vi "Periodic Tasks.vi"(8 "error in":errorcluster) -> ()   [LabVIEW 2020]
doc: "This VI runs in parallel to other tasks. It can contain as many user-defined periodic loops as you need. These can carry out PID or other sorts of timed response."
uses:
  <vilib>/Rock Robotics/WPI/DriverStation/WPI_DriverStationRobotMode2.ctl
  <vilib>/Rock Robotics/WPI/ThirdParty/Phoenix-LabVIEW/Motor Controller/Controls/CTRE_Phoenix_MotorControl_ControlMode.ctl
  <vilib>/Rock Robotics/WPI/Utilities/WPI_GetSetVariantRefNum.vi
  <vilib>/Rock Robotics/Network Tables/NT Write Numeric Array.vi
  Robot Global Data.vi
  <vilib>/Rock Robotics/Network Tables/NT Write Boolean Array.vi
  <vilib>/Rock Robotics/Network Tables/NT Write Boolean.vi
  <vilib>/Rock Robotics/WPI/RobotDrive/WPI_RobotDriveArcadeDrive_Standard(NoSaturation).vi
panel:
  out "Shooter Motor Outtake":bool
  out "Shooter Motor Intake":bool
  out "Conveyor Motor Outtake":bool
  out "Conveyor Motor Intake":bool
  out "Grabber Motor Intake":bool
  out "Grabber Motor Outtake":bool
  out "Slow Speed On":bool
  out "Backwards On":bool
  # "s"
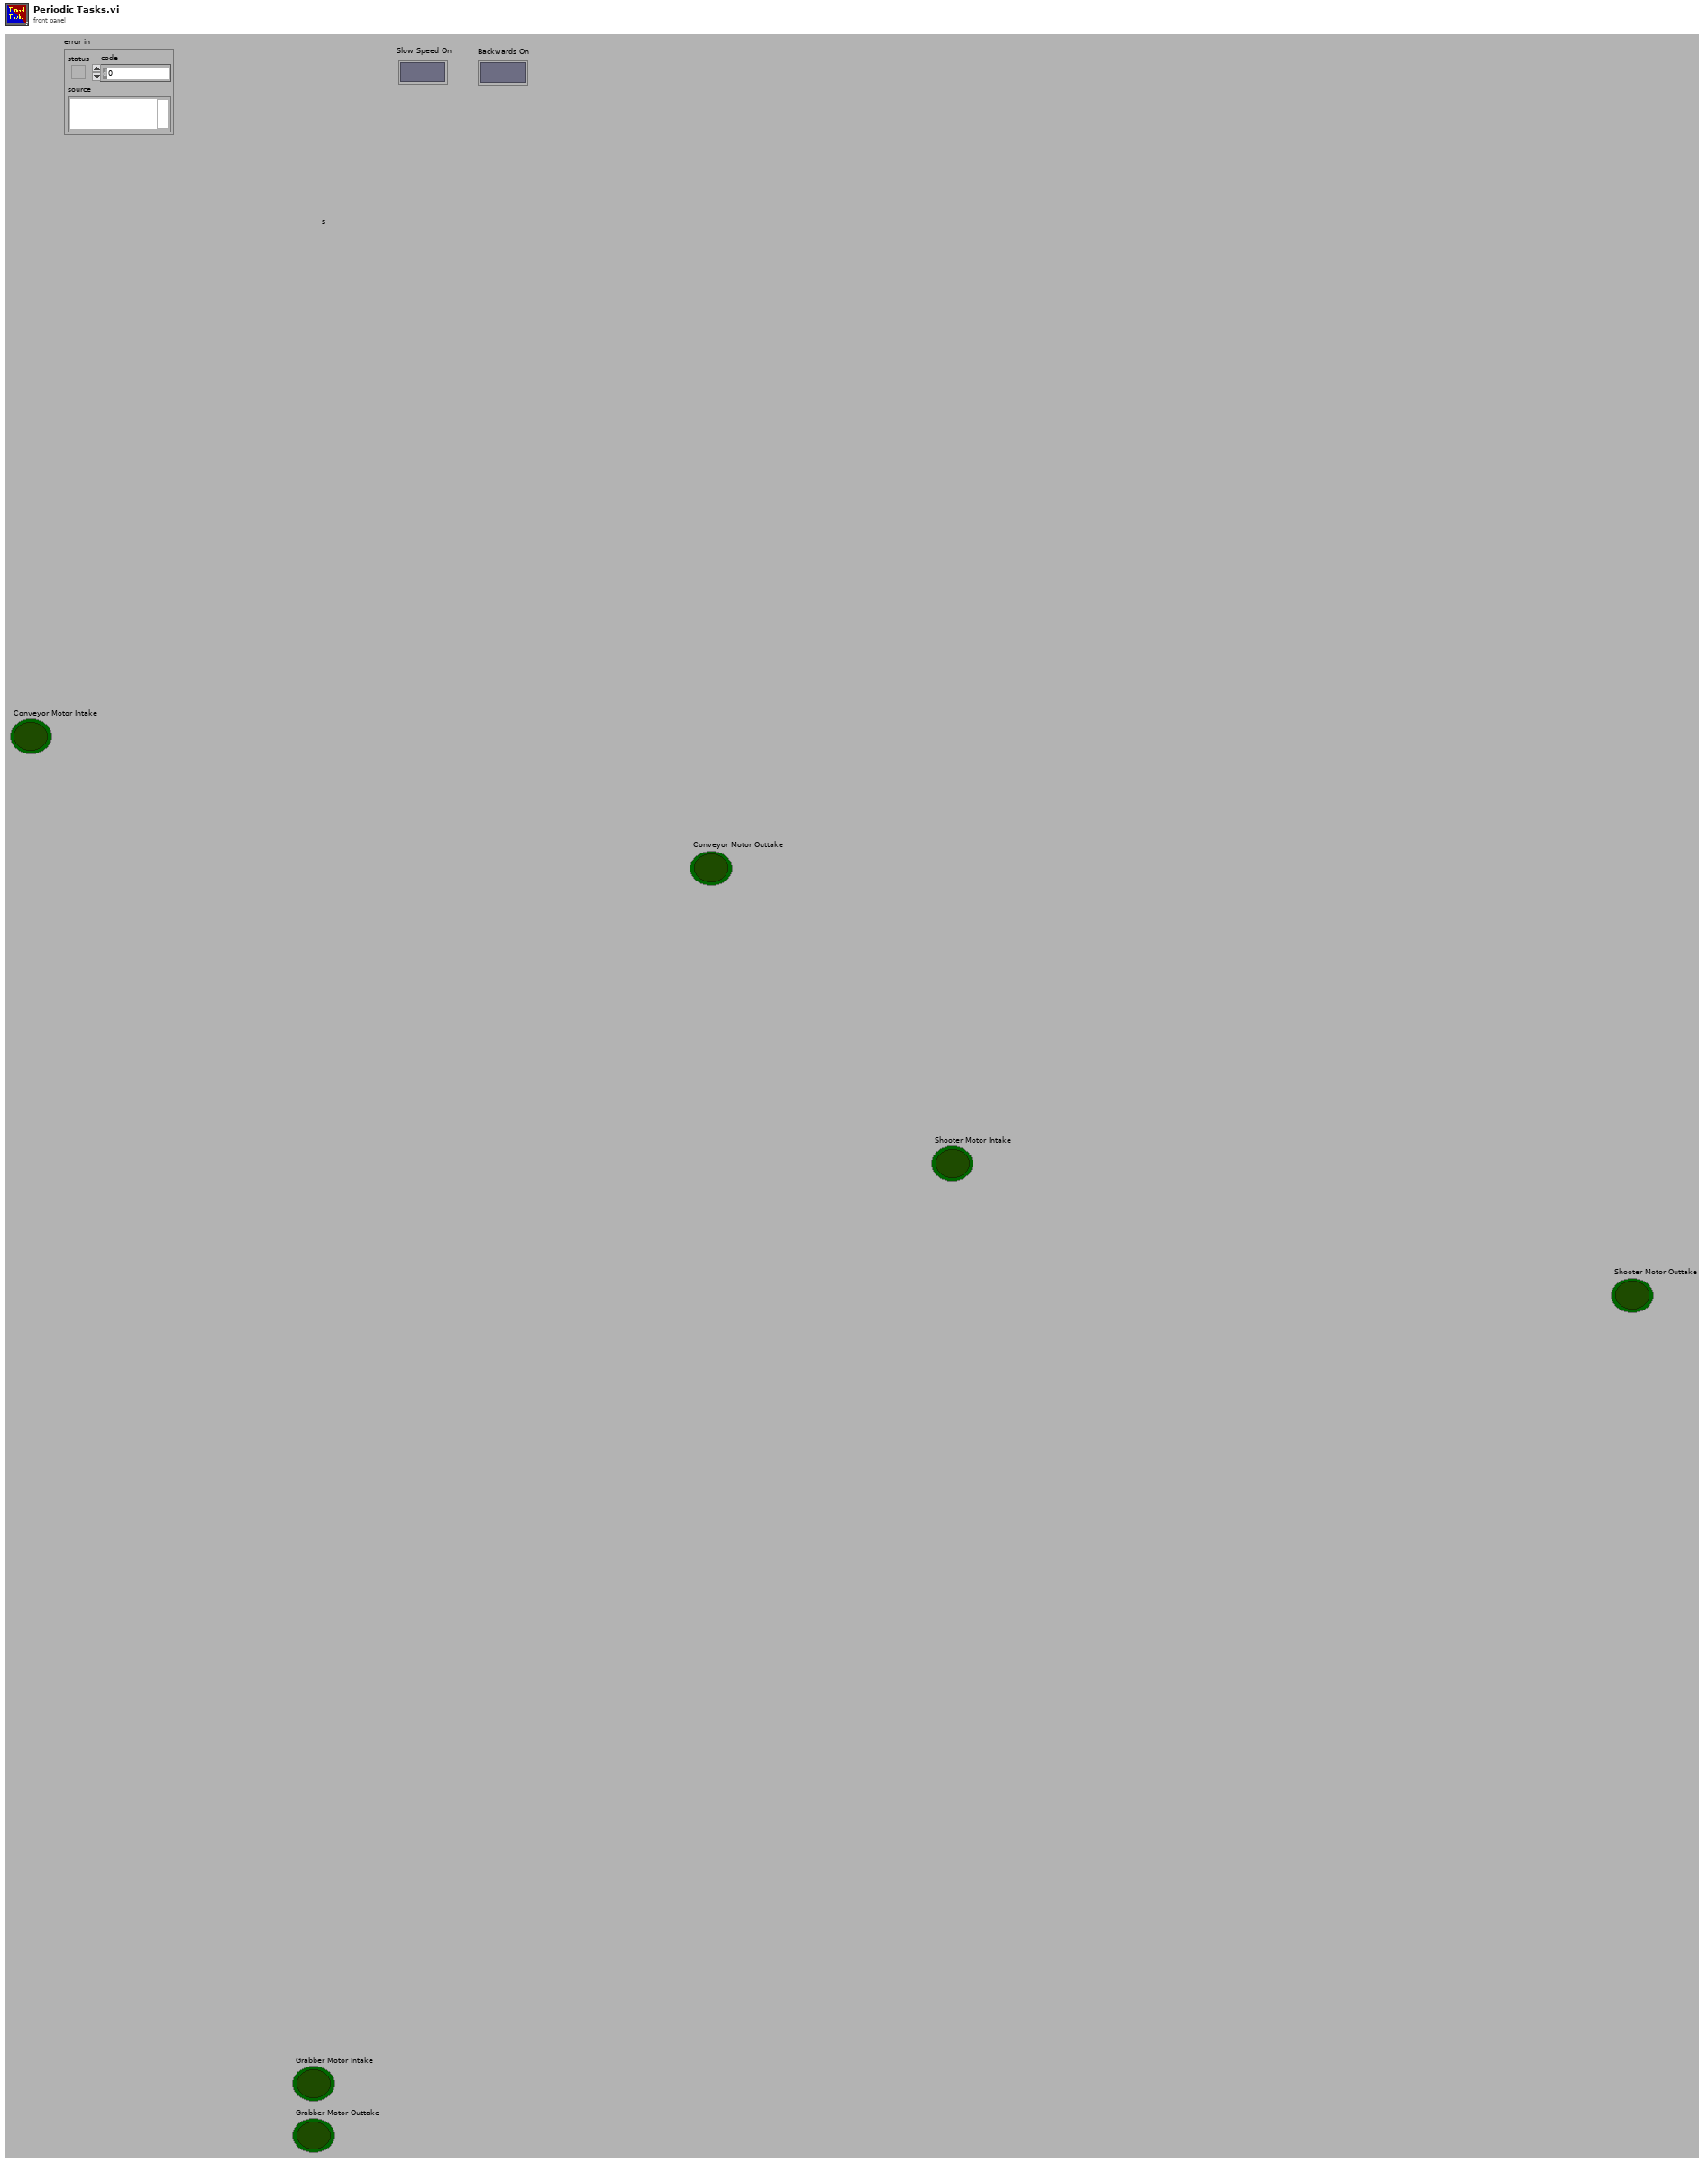
[diagram p1: front panel]
types:
  T1 = typedef "WPI_MotorControlDeviceRef.ctl" = cluster{"DeviceStatus":errorcluster, "Type":T2, "PWM":cluster{"PWM Channel":T3, "DeadBand":T4}, "CAN":cluster{"Device Number":u8, "SetOutput VI Ref":variant, "GetOutput VI Ref":variant, "Enable VI Ref":variant, "Disable VI Ref":variant, "Data":variant}, "Invert":bool, "DIO PWM":cluster{"PWM \"Enable\" Channel":T3, "DIOChannel":T5, "PWM Rate":dbl}}
  T2 = typedef "WPI_MotorControlType.ctl" = enum16{"PWM", "CAN", "DIO PWM"}
  T3 = typedef "FPGA_DIOPWMChannel.ctl" = enum8{"PWM 0", "PWM 1", "PWM 2", "PWM 3", "PWM 4", "PWM 5", "PWM 6", "PWM 7", "PWM 8", "PWM 9", "PWM MXP 0", "PWM MXP 1", "PWM MXP 2", "PWM MXP 3", "PWM MXP 4", "PWM MXP 5", "PWM MXP 6", "PWM MXP 7", "PWM MXP 8", "PWM MXP 9", "Invalid"}
  T4 = typedef "WPI_PWMDeadband.ctl" = cluster{"Name":string, "maxPositivePwm":i32, "minPositivePwm":i32, "centerPwm":i32, "maxNegativePwm":i32, "minNegativePwm":i32, "angularRange":u16}
  T5 = typedef "FPGA_DIOChannel.ctl" = enum8{"DIO 0", "DIO 1", "DIO 2", "DIO 3", "DIO 4", "DIO 5", "DIO 6", "DIO 7", "DIO 8", "DIO 9", "DIO MXP 0", "DIO MXP 1", "DIO MXP 2", "DIO MXP 3", "DIO MXP 4", "DIO MXP 5", "DIO MXP 6", "DIO MXP 7", "DIO MXP 8", "DIO MXP 9", "DIO MXP 10", "DIO MXP 11", "DIO MXP 12", "DIO MXP 13", "DIO MXP 14", "DIO MXP 15", "SPI Port CS1", "SPI Port CS2", "SPI Port CS3", "SPI Port MISO", "SPI Port MOSI", "Invalid"}
  T6 = typedef "WPI_JoystickDevRef.ctl" = cluster{"Device":T7}
  T7 = typedef "WPI_JoystickDeviceEnum.ctl" = enum16{"USB 0", "USB 1", "USB 2", "USB 3", "USB 4", "USB 5"}
  T8 = typedef "WPI_RobotDriveDevRef.ctl" = cluster{"DevStatus":errorcluster, "Motors[]":T1[], "Square Inputs":bool, "Max Output":dbl}
  T9 = typedef "WPI_DriverStationRobotMode2.ctl" = enum16{"Autonomous Disabled", "Autonomous Enabled", "Teleop Disabled", "Teleop Enabled", "Disconnected", "Finish", "Test Disabled", "Test Enabled", "Emergency Stopped"}
  T10 = typedef "CTRE_Phoenix_MotorControl_ControlMode.ctl" = u16
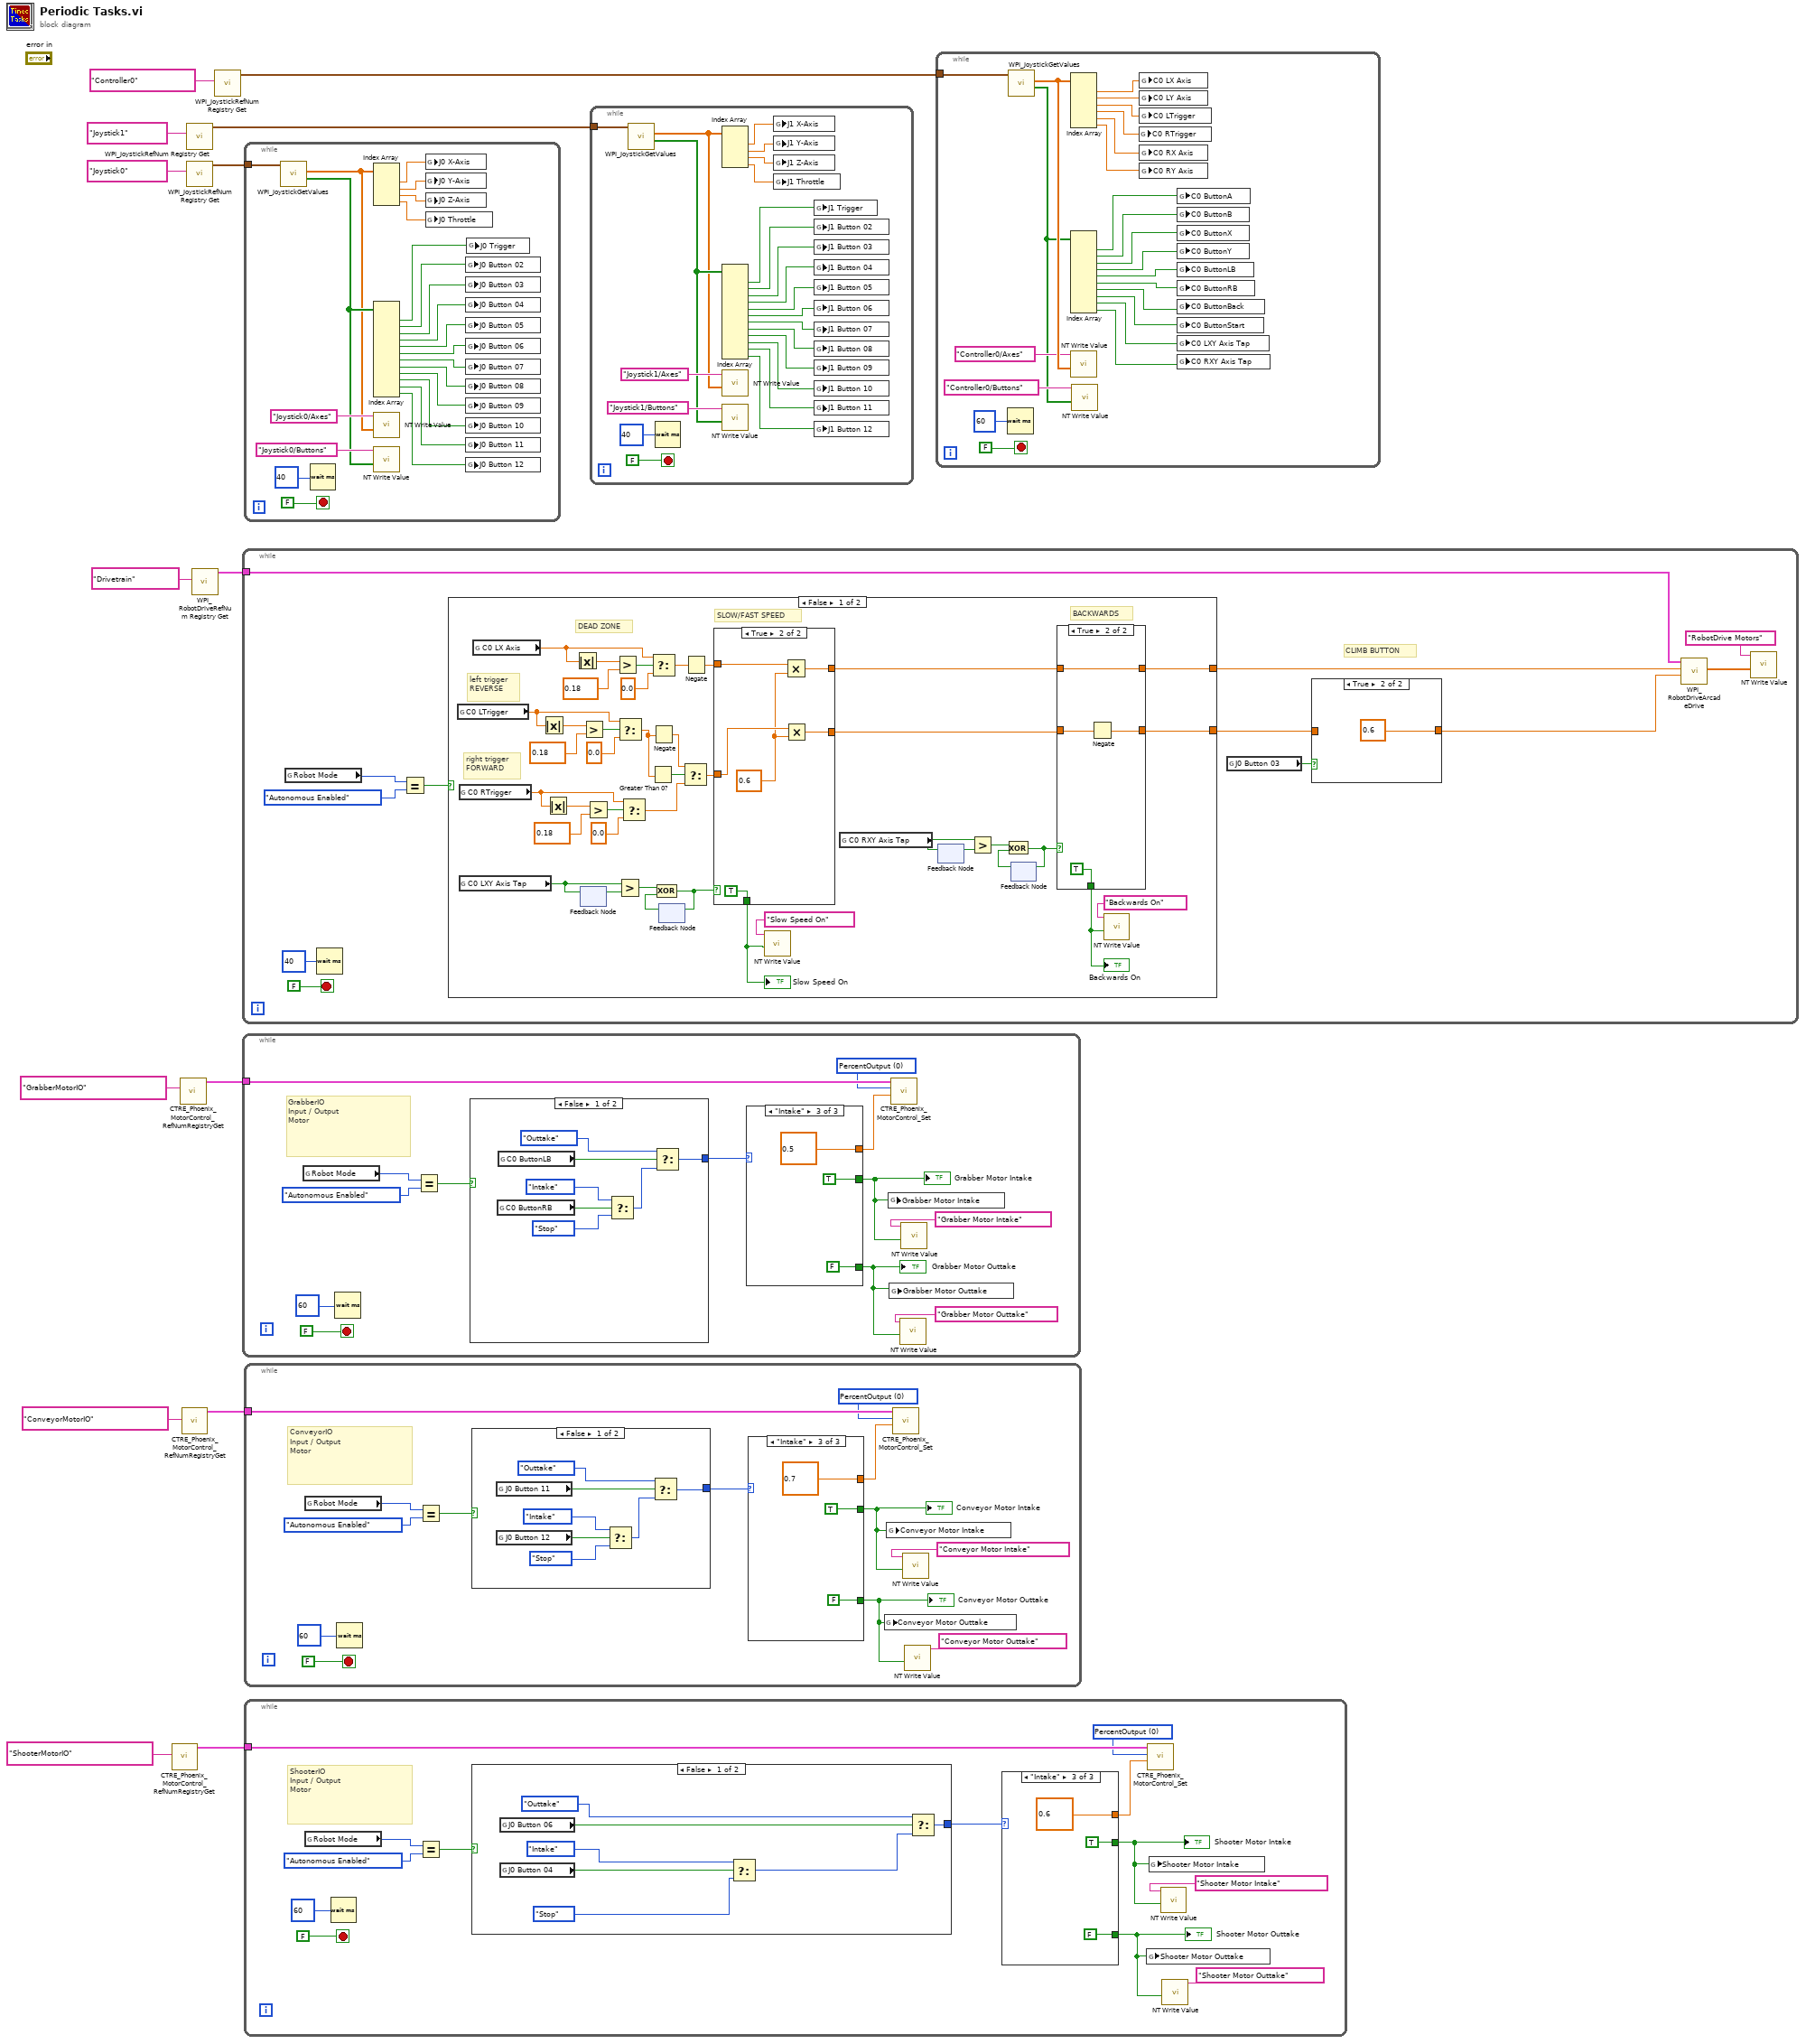
[diagram p0: block diagram]
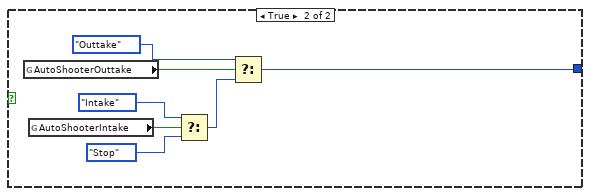
[diagram p2: hidden frame]
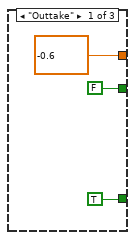
[diagram p3: hidden frame]
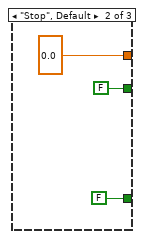
[diagram p4: hidden frame]
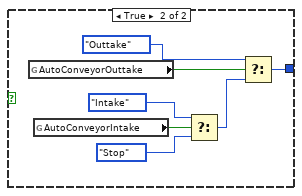
[diagram p5: hidden frame]
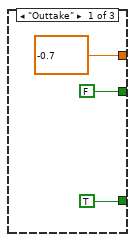
[diagram p6: hidden frame]
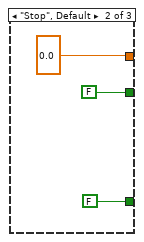
[diagram p7: hidden frame]
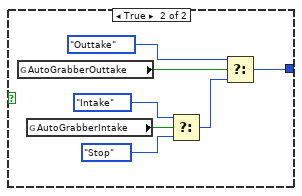
[diagram p8: hidden frame]
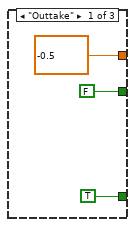
[diagram p9: hidden frame]
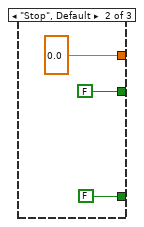
[diagram p10: hidden frame]
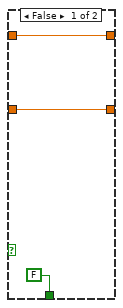
[diagram p12: hidden frame]
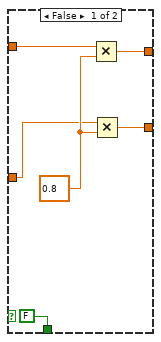
[diagram p13: hidden frame]
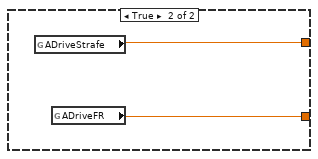
[diagram p14: hidden frame]
diagram:
  n1 = call <vilib>:"CTRE_Phoenix_MotorControl_RefNumRegistryGet.vi"("refnum name"="ShooterMotorIO") -> ("PhoenixMotorControlDevRef"=w2:T1)  [unwired: 9 in, 1 out]
  n2 = call <vilib>:"CTRE_Phoenix_MotorControl_RefNumRegistryGet.vi"("refnum name"="GrabberMotorIO") -> ("PhoenixMotorControlDevRef"=w7:T1)  [unwired: 9 in, 1 out]
  n3 = call <vilib>:"CTRE_Phoenix_MotorControl_RefNumRegistryGet.vi"("refnum name"="ConveyorMotorIO") -> ("PhoenixMotorControlDevRef"=w3:T1)  [unwired: 9 in, 1 out]
  n4 = call <vilib>:"WPI_JoystickRefNum Registry Get.vi"("refnum name"="Joystick1") -> ("JoystickDevRef"=w10:T6)  [unwired: 1 in, 9 out]
  n5 = call <vilib>:"WPI_JoystickRefNum Registry Get.vi"("refnum name"="Joystick0") -> ("JoystickDevRef"=w12:T6)  [unwired: 1 in, 9 out]
  n6 = call <vilib>:"WPI_RobotDriveRefNum Registry Get.vi"("refnum name"="Drivetrain") -> ("RobotDriveDevRef"=w9:T8)  [unwired: 1 in, 9 out]
  n7 = call <vilib>:"WPI_JoystickRefNum Registry Get.vi"("refnum name"="Controller0") -> ("JoystickDevRef"=w5:T6)  [unwired: 1 in, 9 out]
  n8 = while {
    tunnel: w9 -> [w18]
    stop <- FALSE stop-if-true
    # "CLIMB BUTTON"
    n9 = global read "Robot Global Data.vi" "Robot Mode"() -> (w25:T9)
    n10 = Wait (ms)(milliseconds to wait=u32 40) -> ()  [unwired: 1 out]
    n11 = Equal?(x=w25, y=WPI_DriverStationRobotMode2."Autonomous Enabled") -> (x = y?=w23:bool)
    n12 = case shown="False" w23 {
      tunnel: [w43 w88] -> w20
      tunnel: [w42 w89] -> w16
      frame False {
        # "right trigger FORWARD"
        # "left trigger REVERSE"
        # "DEAD ZONE"
        # "BACKWARDS"
        # "SLOW/FAST SPEED"
        n13 = global read "Robot Global Data.vi" "C0 LTrigger"() -> (w53:dbl)
        n14 = global read "Robot Global Data.vi" "C0 RTrigger"() -> (w34:dbl)
        n15 = global read "Robot Global Data.vi" "C0 LXY Axis Tap"() -> (w51:bool)
        n16 = global read "Robot Global Data.vi" "C0 LX Axis"() -> (w54:dbl)
        n17 = Absolute Value(x=w53) -> (abs(x)=w64:dbl)
        n18 = Absolute Value(x=w34) -> (abs(x)=w37:dbl)
        n19 = Absolute Value(x=w54) -> (abs(x)=w62:dbl)
        n20 = feedback #1() -> (w67:bool)  [unwired: 1 in]
        n21 = feedback-in #1(w51) -> ()
        n22 = Greater?(x=w64, y=0.18) -> (0:w65:bool)
        n23 = Greater?(x=w37, y=0.18) -> (0:w38:bool)
        n24 = Greater?(x=w62, y=0.18) -> (0:w63:bool)
        n25 = Select(t=w53, s=w65, f=0.0) -> (s? t:f=w30:dbl)
        n26 = Greater?(x=w51, y=w67) -> (0:w66:bool)
        n27 = Select(t=w34, s=w38, f=0.0) -> (s? t:f=w33:dbl)
        n28 = Greater Than 0?(x=w30) -> (x > 0?=w31:bool)
        n29 = Select(t=w54, s=w63, f=0.0) -> (s? t:f=w40:dbl)
        n30 = Negate(x=w30) -> (-x=w29:dbl)
        n31 = feedback #2() -> (w68:bool)  [unwired: 1 in]
        n32 = Exclusive Or(1:w68, 2:w66) -> (0:w52:bool)
        n33 = feedback-in #2(w52) -> ()
        n34 = Select(t=w29, s=w31, f=w33) -> (s? t:f=w32:dbl)
        n35 = Negate(x=w40) -> (-x=w39:dbl)
        n36 = case shown="True" w52 {
          tunnel: w39 -> [w80 w87]
          tunnel: w32 -> [w79 w86]
          tunnel: [w78 w85] -> w41
          tunnel: [w77 w84] -> w44
          tunnel: [FALSE ("Boolean") TRUE ("Boolean")] -> w50
          frame False {
            w81 = 0.8 ("y")
            n37 = Multiply(x=w80, y=w81) -> (x*y=w78:dbl)
            n38 = Multiply(x=w79, y=w81) -> (x*y=w77:dbl)
          }
          frame True {
            w83 = 0.6 ("y")
            n39 = Multiply(x=w87, y=w83) -> (x*y=w85:dbl)
            n40 = Multiply(x=w86, y=w83) -> (x*y=w84:dbl)
          }
        }
        "Slow Speed On" <- w50
        n41 = call-poly <vilib>:"NT Write Value.vi"("Boolean"=w50, "Name"="Slow Speed On") -> ()  [unwired: 9 in, 1 out]
        n42 = global read "Robot Global Data.vi" "C0 RXY Axis Tap"() -> (w49:bool)
        n43 = feedback #3() -> (w48:bool)  [unwired: 1 in]
        n44 = feedback-in #3(w49) -> ()
        n45 = Greater?(x=w49, y=w48) -> (0:w55:bool)
        n46 = feedback #4() -> (w47:bool)  [unwired: 1 in]
        n47 = Exclusive Or(1:w47, 2:w55) -> (0:w46:bool)
        n48 = feedback-in #4(w46) -> ()
        n49 = case shown="True" w46 {
          tunnel: w44 -> [w70 w74]
          tunnel: w41 -> [w69 w72]
          tunnel: [w70 w73] -> w43
          tunnel: [w69 w72] -> w42
          tunnel: [FALSE ("Boolean") TRUE ("Boolean")] -> w45
          frame False {
          }
          frame True {
            n50 = Negate(x=w74) -> (-x=w73:dbl)
          }
        }
        "Backwards On" <- w45
        n51 = call-poly <vilib>:"NT Write Value.vi"("Boolean"=w45, "Name"="Backwards On") -> ()  [unwired: 9 in, 1 out]
      }
      frame True {
        n52 = global read "Robot Global Data.vi" "ADriveStrafe"() -> (w89:dbl)
        n53 = global read "Robot Global Data.vi" "ADriveFR"() -> (w88:dbl)
      }
    }
    n54 = global read "Robot Global Data.vi" "J0 Button 03"() -> (w19:bool)
    n55 = case shown="True" w19 {
      tunnel: w20 -> [w27 _]
      tunnel: [w27 0.6 ("y")] -> w15
      frame False {
      }
      frame True {
      }
    }
    n56 = call-poly <vilib>:"WPI_RobotDriveArcadeDrive.vi"("Y axis value"=w15, "X axis value"=w16, "RobotDriveDevRef"=w18) -> ("Motor Values"=w17:dbl[])  [unwired: 6 in, 2 out]
    n57 = call-poly <vilib>:"NT Write Value.vi"("Numeric Array"=w17, "Name"="RobotDrive Motors") -> ()  [unwired: 9 in, 1 out]
  }
  n58 = while {
    tunnel: w7 -> [w99]
    stop <- FALSE stop-if-true
    w94 = T10 0 items=["PercentOutput"=0, "Position"=1, "Velocity"=2, "Current"=3, "Follower"=5, "MotionProfile"=6, "MotionMagic"=7, "MotionProfileArc"=10, "Disabled"=15] ("Control Mode")
    # "GrabberIO\nInput / Output\nMotor"
    n59 = global read "Robot Global Data.vi" "Robot Mode"() -> (w98:T9)
    n60 = Wait (ms)(milliseconds to wait=u32 60) -> ()  [unwired: 1 out]
    n61 = Equal?(x=w98, y=WPI_DriverStationRobotMode2."Autonomous Enabled") -> (x = y?=w96:bool)
    n62 = case shown="False" w96 {
      tunnel: [w105 w110] -> w95
      frame False {
        n63 = global read "Robot Global Data.vi" "C0 ButtonRB"() -> (w103:bool)
        n64 = global read "Robot Global Data.vi" "C0 ButtonLB"() -> (w104:bool)
        n65 = Select(t=enum16{"Outtake", "Intake", "Stop"}."Intake", s=w103, f=enum16{"Outtake", "Intake", "Stop"}."Stop") -> (s? t:f=w106:enum16{"Outtake", "Intake", "Stop"})
        n66 = Select(t=enum16{"Outtake", "Intake", "Stop"}."Outtake", s=w104, f=w106) -> (s? t:f=w105:enum16{"Outtake", "Intake", "Stop"})
      }
      frame True {
        n67 = global read "Robot Global Data.vi" "AutoGrabberOuttake"() -> (w112:bool)
        n68 = global read "Robot Global Data.vi" "AutoGrabberIntake"() -> (w114:bool)
        n69 = Select(t=enum16{"Outtake", "Intake", "Stop"}."Intake", s=w114, f=enum16{"Outtake", "Intake", "Stop"}."Stop") -> (s? t:f=w111:enum16{"Outtake", "Intake", "Stop"})
        n70 = Select(t=enum16{"Outtake", "Intake", "Stop"}."Outtake", s=w112, f=w111) -> (s? t:f=w110:enum16{"Outtake", "Intake", "Stop"})
      }
    }
    n71 = case shown="\"Intake\"" w95 {
      tunnel: [-0.5 0.0 0.5] -> w100
      tunnel: [FALSE FALSE TRUE] -> w90
      tunnel: [TRUE FALSE FALSE] -> w91
      frame "Outtake" {
      }
      frame "Stop", Default {
      }
      frame "Intake" {
      }
    }
    "Grabber Motor Intake" <- w90
    "Grabber Motor Outtake" <- w91
    n72 = global write "Robot Global Data.vi" "Grabber Motor Intake"(w90) -> ()
    n73 = global write "Robot Global Data.vi" "Grabber Motor Outtake"(w91) -> ()
    n74 = call <vilib>:"CTRE_Phoenix_MotorControl_Set.vi"("Output"=w100, "Control Mode"=w94, "PhoenixMotorControlDevRef"=w99) -> ()  [unwired: 7 in, 2 out]
    n75 = call-poly <vilib>:"NT Write Value.vi"("Boolean"=w91, "Name"="Grabber Motor Outtake") -> ()  [unwired: 9 in, 1 out]
    n76 = call-poly <vilib>:"NT Write Value.vi"("Boolean"=w90, "Name"="Grabber Motor Intake") -> ()  [unwired: 9 in, 1 out]
  }
  n77 = while {
    tunnel: w12 -> [w146]
    stop <- FALSE stop-if-true
    n78 = call <vilib>:"WPI_JoystickGetValues.vi"("JoystickDevRef"=w146) -> ("Buttons"=w127:bool[], "Axes"=w126:dbl[])  [unwired: 6 in, 3 out]
    n79 = Wait (ms)(milliseconds to wait=u32 40) -> ()  [unwired: 1 out]
    n80 = Index Array(array=w126) -> (element #1=w145:dbl, element #2=w144:dbl, element #3=w143:dbl, element #4=w142:dbl)  [unwired: 4 in]
    n81 = Index Array(array=w127) -> (element #1=w141:bool, element #2=w140:bool, element #3=w139:bool, element #4=w138:bool, element #5=w137:bool, element #6=w136:bool, element #7=w135:bool, element #8=w134:bool, element #9=w133:bool, element #10=w132:bool, element #11=w131:bool, element #12=w130:bool)  [unwired: 12 in]
    n82 = call-poly <vilib>:"NT Write Value.vi"("Numeric Array"=w126, "Name"="Joystick0/Axes") -> ()  [unwired: 9 in, 1 out]
    n83 = call-poly <vilib>:"NT Write Value.vi"("Boolean Array"=w127, "Name"="Joystick0/Buttons") -> ()  [unwired: 9 in, 1 out]
    n84 = global write "Robot Global Data.vi" "J0 X-Axis"(w145) -> ()
    n85 = global write "Robot Global Data.vi" "J0 Y-Axis"(w144) -> ()
    n86 = global write "Robot Global Data.vi" "J0 Z-Axis"(w143) -> ()
    n87 = global write "Robot Global Data.vi" "J0 Throttle"(w142) -> ()
    n88 = global write "Robot Global Data.vi" "J0 Button 02"(w140) -> ()
    n89 = global write "Robot Global Data.vi" "J0 Button 03"(w139) -> ()
    n90 = global write "Robot Global Data.vi" "J0 Button 04"(w138) -> ()
    n91 = global write "Robot Global Data.vi" "J0 Button 05"(w137) -> ()
    n92 = global write "Robot Global Data.vi" "J0 Button 06"(w136) -> ()
    n93 = global write "Robot Global Data.vi" "J0 Button 07"(w135) -> ()
    n94 = global write "Robot Global Data.vi" "J0 Button 08"(w134) -> ()
    n95 = global write "Robot Global Data.vi" "J0 Button 09"(w133) -> ()
    n96 = global write "Robot Global Data.vi" "J0 Button 10"(w132) -> ()
    n97 = global write "Robot Global Data.vi" "J0 Button 11"(w131) -> ()
    n98 = global write "Robot Global Data.vi" "J0 Button 12"(w130) -> ()
    n99 = global write "Robot Global Data.vi" "J0 Trigger"(w141) -> ()
  }
  n100 = while {
    tunnel: w3 -> [w158]
    stop <- FALSE stop-if-true
    w153 = T10 0 items=["PercentOutput"=0, "Position"=1, "Velocity"=2, "Current"=3, "Follower"=5, "MotionProfile"=6, "MotionMagic"=7, "MotionProfileArc"=10, "Disabled"=15] ("Control Mode")
    # "ConveyorIO\nInput / Output\nMotor"
    n101 = global read "Robot Global Data.vi" "Robot Mode"() -> (w157:T9)
    n102 = Wait (ms)(milliseconds to wait=u32 60) -> ()  [unwired: 1 out]
    n103 = Equal?(x=w157, y=WPI_DriverStationRobotMode2."Autonomous Enabled") -> (x = y?=w155:bool)
    n104 = case shown="False" w155 {
      tunnel: [w162 w169] -> w154
      frame False {
        n105 = global read "Robot Global Data.vi" "J0 Button 11"() -> (w164:bool)
        n106 = global read "Robot Global Data.vi" "J0 Button 12"() -> (w166:bool)
        n107 = Select(t=enum16{"Outtake", "Intake", "Stop"}."Intake", s=w166, f=enum16{"Outtake", "Intake", "Stop"}."Stop") -> (s? t:f=w163:enum16{"Outtake", "Intake", "Stop"})
        n108 = Select(t=enum16{"Outtake", "Intake", "Stop"}."Outtake", s=w164, f=w163) -> (s? t:f=w162:enum16{"Outtake", "Intake", "Stop"})
      }
      frame True {
        n109 = global read "Robot Global Data.vi" "AutoConveyorOuttake"() -> (w171:bool)
        n110 = global read "Robot Global Data.vi" "AutoConveyorIntake"() -> (w173:bool)
        n111 = Select(t=enum16{"Outtake", "Intake", "Stop"}."Intake", s=w173, f=enum16{"Outtake", "Intake", "Stop"}."Stop") -> (s? t:f=w170:enum16{"Outtake", "Intake", "Stop"})
        n112 = Select(t=enum16{"Outtake", "Intake", "Stop"}."Outtake", s=w171, f=w170) -> (s? t:f=w169:enum16{"Outtake", "Intake", "Stop"})
      }
    }
    n113 = case shown="\"Intake\"" w154 {
      tunnel: [-0.7 0.0 0.7] -> w159
      tunnel: [FALSE FALSE TRUE] -> w149
      tunnel: [TRUE FALSE FALSE] -> w150
      frame "Outtake" {
      }
      frame "Stop", Default {
      }
      frame "Intake" {
      }
    }
    "Conveyor Motor Intake" <- w149
    "Conveyor Motor Outtake" <- w150
    n114 = global write "Robot Global Data.vi" "Conveyor Motor Outtake"(w150) -> ()
    n115 = global write "Robot Global Data.vi" "Conveyor Motor Intake"(w149) -> ()
    n116 = call <vilib>:"CTRE_Phoenix_MotorControl_Set.vi"("Output"=w159, "Control Mode"=w153, "PhoenixMotorControlDevRef"=w158) -> ()  [unwired: 7 in, 2 out]
    n117 = call-poly <vilib>:"NT Write Value.vi"("Boolean"=w149, "Name"="Conveyor Motor Intake") -> ()  [unwired: 9 in, 1 out]
    n118 = call-poly <vilib>:"NT Write Value.vi"("Boolean"=w150, "Name"="Conveyor Motor Outtake") -> ()  [unwired: 9 in, 1 out]
  }
  n119 = while {
    tunnel: w2 -> [w194]
    stop <- FALSE stop-if-true
    w189 = T10 0 items=["PercentOutput"=0, "Position"=1, "Velocity"=2, "Current"=3, "Follower"=5, "MotionProfile"=6, "MotionMagic"=7, "MotionProfileArc"=10, "Disabled"=15] ("Control Mode")
    # "ShooterIO\nInput / Output\nMotor"
    n120 = global read "Robot Global Data.vi" "Robot Mode"() -> (w193:T9)
    n121 = Wait (ms)(milliseconds to wait=u32 60) -> ()  [unwired: 1 out]
    n122 = Equal?(x=w193, y=WPI_DriverStationRobotMode2."Autonomous Enabled") -> (x = y?=w191:bool)
    n123 = case shown="False" w191 {
      tunnel: [w200 w205] -> w190
      frame False {
        n124 = global read "Robot Global Data.vi" "J0 Button 06"() -> (w198:bool)
        n125 = global read "Robot Global Data.vi" "J0 Button 04"() -> (w199:bool)
        n126 = Select(t=enum16{"Outtake", "Intake", "Stop"}."Intake", s=w199, f=enum16{"Outtake", "Intake", "Stop"}."Stop") -> (s? t:f=w201:enum16{"Outtake", "Intake", "Stop"})
        n127 = Select(t=enum16{"Outtake", "Intake", "Stop"}."Outtake", s=w198, f=w201) -> (s? t:f=w200:enum16{"Outtake", "Intake", "Stop"})
      }
      frame True {
        n128 = global read "Robot Global Data.vi" "AutoShooterOuttake"() -> (w207:bool)
        n129 = global read "Robot Global Data.vi" "AutoShooterIntake"() -> (w209:bool)
        n130 = Select(t=enum16{"Outtake", "Intake", "Stop"}."Intake", s=w209, f=enum16{"Outtake", "Intake", "Stop"}."Stop") -> (s? t:f=w206:enum16{"Outtake", "Intake", "Stop"})
        n131 = Select(t=enum16{"Outtake", "Intake", "Stop"}."Outtake", s=w207, f=w206) -> (s? t:f=w205:enum16{"Outtake", "Intake", "Stop"})
      }
    }
    n132 = case shown="\"Intake\"" w190 {
      tunnel: [-0.6 0.0 0.6] -> w195
      tunnel: [FALSE FALSE TRUE] -> w185
      tunnel: [TRUE FALSE FALSE] -> w186
      frame "Outtake" {
      }
      frame "Stop", Default {
      }
      frame "Intake" {
      }
    }
    "Shooter Motor Intake" <- w185
    "Shooter Motor Outtake" <- w186
    n133 = global write "Robot Global Data.vi" "Shooter Motor Outtake"(w186) -> ()
    n134 = call <vilib>:"CTRE_Phoenix_MotorControl_Set.vi"("Output"=w195, "Control Mode"=w189, "PhoenixMotorControlDevRef"=w194) -> ()  [unwired: 7 in, 2 out]
    n135 = global write "Robot Global Data.vi" "Shooter Motor Intake"(w185) -> ()
    n136 = call-poly <vilib>:"NT Write Value.vi"("Boolean"=w185, "Name"="Shooter Motor Intake") -> ()  [unwired: 9 in, 1 out]
    n137 = call-poly <vilib>:"NT Write Value.vi"("Boolean"=w186, "Name"="Shooter Motor Outtake") -> ()  [unwired: 9 in, 1 out]
  }
  n138 = while {
    tunnel: w10 -> [w241]
    stop <- FALSE stop-if-true
    n139 = call <vilib>:"WPI_JoystickGetValues.vi"("JoystickDevRef"=w241) -> ("Buttons"=w222:bool[], "Axes"=w221:dbl[])  [unwired: 6 in, 3 out]
    n140 = Wait (ms)(milliseconds to wait=u32 40) -> ()  [unwired: 1 out]
    n141 = Index Array(array=w221) -> (element #1=w240:dbl, element #2=w239:dbl, element #3=w238:dbl, element #4=w237:dbl)  [unwired: 4 in]
    n142 = Index Array(array=w222) -> (element #1=w236:bool, element #2=w235:bool, element #3=w234:bool, element #4=w233:bool, element #5=w232:bool, element #6=w231:bool, element #7=w230:bool, element #8=w229:bool, element #9=w228:bool, element #10=w227:bool, element #11=w226:bool, element #12=w225:bool)  [unwired: 12 in]
    n143 = call-poly <vilib>:"NT Write Value.vi"("Numeric Array"=w221, "Name"="Joystick1/Axes") -> ()  [unwired: 9 in, 1 out]
    n144 = call-poly <vilib>:"NT Write Value.vi"("Boolean Array"=w222, "Name"="Joystick1/Buttons") -> ()  [unwired: 9 in, 1 out]
    n145 = global write "Robot Global Data.vi" "J1 X-Axis"(w240) -> ()
    n146 = global write "Robot Global Data.vi" "J1 Y-Axis"(w239) -> ()
    n147 = global write "Robot Global Data.vi" "J1 Z-Axis"(w238) -> ()
    n148 = global write "Robot Global Data.vi" "J1 Throttle"(w237) -> ()
    n149 = global write "Robot Global Data.vi" "J1 Trigger"(w236) -> ()
    n150 = global write "Robot Global Data.vi" "J1 Button 02"(w235) -> ()
    n151 = global write "Robot Global Data.vi" "J1 Button 03"(w234) -> ()
    n152 = global write "Robot Global Data.vi" "J1 Button 04"(w233) -> ()
    n153 = global write "Robot Global Data.vi" "J1 Button 05"(w232) -> ()
    n154 = global write "Robot Global Data.vi" "J1 Button 06"(w231) -> ()
    n155 = global write "Robot Global Data.vi" "J1 Button 07"(w230) -> ()
    n156 = global write "Robot Global Data.vi" "J1 Button 08"(w229) -> ()
    n157 = global write "Robot Global Data.vi" "J1 Button 09"(w228) -> ()
    n158 = global write "Robot Global Data.vi" "J1 Button 10"(w227) -> ()
    n159 = global write "Robot Global Data.vi" "J1 Button 11"(w226) -> ()
    n160 = global write "Robot Global Data.vi" "J1 Button 12"(w225) -> ()
  }
  n161 = while {
    tunnel: w5 -> [w261]
    stop <- FALSE stop-if-true
    n162 = Wait (ms)(milliseconds to wait=u32 60) -> ()  [unwired: 1 out]
    n163 = call <vilib>:"WPI_JoystickGetValues.vi"("JoystickDevRef"=w261) -> ("Buttons"=w256:bool[], "Axes"=w263:dbl[])  [unwired: 6 in, 3 out]
    n164 = Index Array(array=w263) -> (element #1=w260:dbl, element #2=w259:dbl, element #3=w258:dbl, element #4=w248:dbl, element #5=w247:dbl, element #6=w246:dbl)  [unwired: 6 in]
    n165 = Index Array(array=w256) -> (element #1=w257:bool, element #2=w244:bool, element #3=w255:bool, element #4=w254:bool, element #5=w245:bool, element #6=w253:bool, element #7=w252:bool, element #8=w251:bool, element #9=w250:bool, element #10=w249:bool)  [unwired: 10 in]
    n166 = call-poly <vilib>:"NT Write Value.vi"("Numeric Array"=w263, "Name"="Controller0/Axes") -> ()  [unwired: 9 in, 1 out]
    n167 = call-poly <vilib>:"NT Write Value.vi"("Boolean Array"=w256, "Name"="Controller0/Buttons") -> ()  [unwired: 9 in, 1 out]
    n168 = global write "Robot Global Data.vi" "C0 RTrigger"(w248) -> ()
    n169 = global write "Robot Global Data.vi" "C0 LX Axis"(w260) -> ()
    n170 = global write "Robot Global Data.vi" "C0 LY Axis"(w259) -> ()
    n171 = global write "Robot Global Data.vi" "C0 LTrigger"(w258) -> ()
    n172 = global write "Robot Global Data.vi" "C0 RX Axis"(w247) -> ()
    n173 = global write "Robot Global Data.vi" "C0 RY Axis"(w246) -> ()
    n174 = global write "Robot Global Data.vi" "C0 ButtonA"(w257) -> ()
    n175 = global write "Robot Global Data.vi" "C0 ButtonB"(w244) -> ()
    n176 = global write "Robot Global Data.vi" "C0 ButtonX"(w255) -> ()
    n177 = global write "Robot Global Data.vi" "C0 ButtonY"(w254) -> ()
    n178 = global write "Robot Global Data.vi" "C0 ButtonLB"(w245) -> ()
    n179 = global write "Robot Global Data.vi" "C0 ButtonRB"(w253) -> ()
    n180 = global write "Robot Global Data.vi" "C0 ButtonBack"(w252) -> ()
    n181 = global write "Robot Global Data.vi" "C0 ButtonStart"(w251) -> ()
    n182 = global write "Robot Global Data.vi" "C0 LXY Axis Tap"(w250) -> ()
    n183 = global write "Robot Global Data.vi" "C0 RXY Axis Tap"(w249) -> ()
  }
